vi "Count Monitor Data.vi"(10 "Monitor Data Cluster in":T1, 11 "Start or Stop Enable?":bool) -> (2 "Monitor Data Cluster out":T1, 3 "Enable?":bool)   [LabVIEW 2016]
uses:
  Typedefs/Monitor Data Cluster.ctl
  <vilib>/rvi/Emulation/niFpgaEmulationIsFPGAContextNoSignature.vi
  <vilib>/rvi/DataTransferAndStorage/Container/Common/niFpgaContainerGetUniqueNameForEmu.vi
  <vilib>/rvi/Memory/Memory_Emulation/niFpgaMemoryEmulationCacheClearOnFirstRun.vi
  <vilib>/rvi/Memory/Memory_Emulation/nirvimemoryEmulationManagerCache_MakeExclusive.vi
  <vilib>/rvi/Memory/Memory_Emulation/niFpgaMemoryEmulationValidateCache.vi
  <vilib>/rvi/Memory/Memory_Emulation/nirvimemoryEmulationManagerCache_InsertValue.vi
  <vilib>/Utility/error.llb/Clear Errors.vi
  <vilib>/rvi/Memory/Memory_Emulation/nirvimemoryEmulationManagerCache_ReleaseExclusive.vi
  <vilib>/rvi/Memory/Memory_Emulation/nirvimemoryEmulationManagerCache_GetValue.vi
  <vilib>/rvi/Memory/Memory_Emulation/nirvimemoryEmulationManagerCache_SetValue.vi
  <vilib>/rvi/Emulation/niFpgaProcessEmulError.vi
  <vilib>/rvi/Emulation/niFpgaSctlEmulationGetInTimedLoop.vi
  <vilib>/rvi/eio/common/nirviEmuTemplateMethod_errors.vi
  <vilib>/rvi/DataTransferAndStorage/Container/XNode/niFpgaContainer.xnode
  <vilib>/rvi/DataTransferAndStorage/Register/Emulation/niFpgaRegisterEmulation.vi
  <vilib>/eio/EIONode/EIONode.xnode
  Host/Typedefs/IO Buffer Operation.ctl
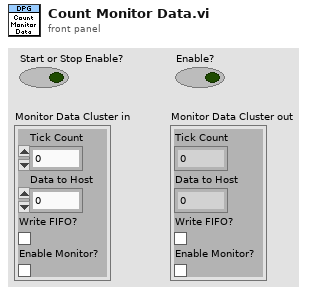
[diagram p1: front panel]
types:
  T1 = typedef "Monitor Data Cluster.ctl" = cluster{"Tick Count":u32, "Data to Host":u64, "Write FIFO?":bool, "Enable Monitor?":bool}
  T2 = typedef "IO Buffer Operation.ctl" = enum16{"Initialize", "Write IO Data_Rd", "Read IO Data_Rd", "Write IO Data_Wr", "Read IO Data_Wr", "Write  IO Data_Dir", "Read  IO Data_Dir", "Write Host to Target FIFO", "Read Host to Target FIFO", "Write Target to Host FIFO", "Read Target to Host FIFO", "Write Monitor Enable?", "Read Monitor Enable?", "Close"}
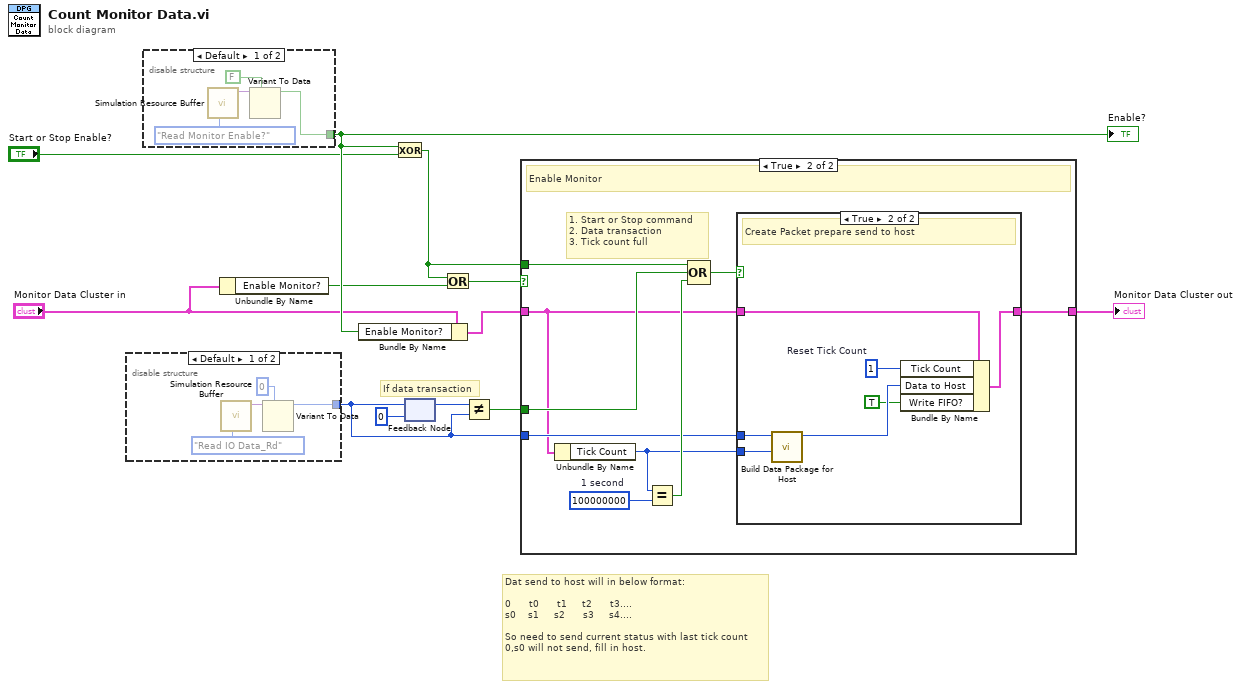
[diagram p0: block diagram]
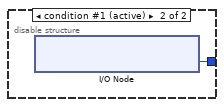
[diagram p2: hidden frame]
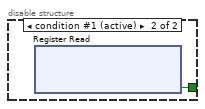
[diagram p3: hidden frame]
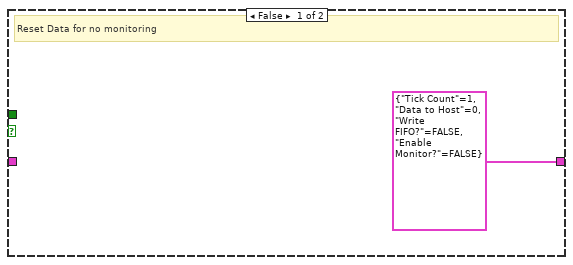
[diagram p4: hidden frame]
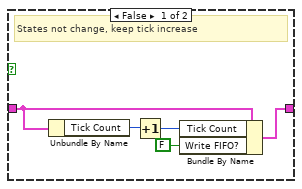
[diagram p5: hidden frame]
diagram:
  # "Dat send to host will in below format:\n\n0\t     t0\t     t1\t    t2\t\t    t3....\ns0\t   s1\t    s2\t     s3\t    s4....\n\nSo need to send current status with last tick count\n0,s0 will not send, fill in host."
  # "If data transaction"
  n1 = disable-structure shown="Default" {
    disable-tunnel: [w14 w17] -> w4
    frame condition #0 {
      n2 = call "Simulation Resource Buffer.vi"("IO Buffer Operation"=IO_Buffer_Operation."Read IO Data_Rd") -> ("Data out"=w16:variant)  [unwired: 8 in, 2 out]
      n3 = Variant To Data(type=u32 0 ("IO Module\\SE_Data_Rd"), Variant=w16) -> (data=w14:u32)  [unwired: 1 in, 1 out]
    }
    frame condition #1 (active) {
      n4 = xnode "I/O Node"() -> ("IO Module\\SE_Data_Rd"=w17:u32)  [unwired: 1 in, 1 out]
    }
  }
  n5 = disable-structure shown="Default" {
    disable-tunnel: [w19 w22] -> w11
    frame condition #0 {
      n6 = call "Simulation Resource Buffer.vi"("IO Buffer Operation"=IO_Buffer_Operation."Read Monitor Enable?") -> ("Data out"=w20:variant)  [unwired: 8 in, 2 out]
      n7 = Variant To Data(type=FALSE ("Start or Stop Enable?"), Variant=w20) -> (data=w19:bool)  [unwired: 1 in, 1 out]
    }
    frame condition #1 (active) {
      n8 = xnode ("Register Read")() -> ("Data"=w22:bool)  [unwired: 1 in, 1 out]
    }
  }
  "Enable?" <- w11
  n9 = Unbundle By Name("Monitor Data Cluster in") -> ("Enable Monitor?"=w10:bool)
  n10 = Bundle By Name(cluster="Monitor Data Cluster in", "Enable Monitor?"=w11) -> (w9:T1)
  n11 = Exclusive Or(1:"Start or Stop Enable?", 2:w11) -> (0:w12:bool)
  n12 = feedback #1(u32 0 ("IO Module\\SE_Data_Rd")) -> (w3:u32)
  n13 = feedback-in #1(w4) -> ()
  n14 = Or(x=w12, y=w10) -> (x .or. y?=w5:bool)
  n15 = Not Equal?(x=w3, y=w4) -> (x != y?=w2:bool)
  n16 = case shown="True" w5 {
    tunnel: w2 -> [_ w30]
    tunnel: w12 -> [_ w31]
    tunnel: w4 -> [_ w27]
    tunnel: w9 -> [_ w25]
    tunnel: [T1 {"Tick Count"=1, "Data to Host"=0, "Write FIFO?"=FALSE, "Enable Monitor?"=FALSE} ("Monitor Data Cluster") w26] -> w6
    frame False {
      # "Reset Data for no monitoring"
    }
    frame True {
      w32 = u32 100000000  # 1 second
      # "1. Start or Stop command \n2. Data transaction\n3. Tick count full"
      # "Enable Monitor"
      n17 = Unbundle By Name(w25) -> ("Tick Count"=w24:u32)
      n18 = Equal?(x=w24, y=w32) -> (x = y?=w29:bool)
      n19 = Compound Arithmetic op=OR(w31, w30, w29) -> (w28:bool)
      n20 = case shown="True" w28 {
        tunnel: w27 -> [_ w44]
        tunnel: w24 -> [_ w43]
        tunnel: w25 -> [w37 w42]
        tunnel: [w34 w41] -> w26
        frame False {
          # "States not change, keep tick increase"
          n21 = Unbundle By Name(w37) -> ("Tick Count"=w36:u32)
          n22 = Increment(x=w36) -> (x+1=w35:u32)
          n23 = Bundle By Name(cluster=w37, "Tick Count"=w35, "Write FIFO?"=FALSE) -> (w34:T1)
        }
        frame True {
          w40 = u32 1  # Reset Tick Count
          # "Create Packet prepare send to host"
          n24 = call "Build Data Package for Host.vi"("Tick Number(U32)"=w43, "IO States(U32)"=w44) -> ("Data to Host (U64)"=w39:u64)  [unwired: 9 in]
          n25 = Bundle By Name(cluster=w42, "Tick Count"=w40, "Data to Host"=w39, "Write FIFO?"=TRUE) -> (w41:T1)
        }
      }
    }
  }
  "Monitor Data Cluster out" <- w6
